vi "ExCamApp.vi"() -> ()   [LabVIEW 2010]
uses:
  MaxY.vi
  MaxX.vi
  temperture.vi
  Binning.vi
  ADC.vi
  readoutport.vi
panel:
  out "Boolean":bool
  in  "Leave Program":bool
  in  "Tab Control":T1(tab)
  out "Pixel Time":i32
  out "Bit Depth":i32
  out "ReadOut port":i32
  out "ADC Offset":i32
  out "ADC Gain":i32
  out "ADC Speed":i32
  in  "Set Controller Variables":bool
  in  "Readout Port":bool
  in  "Gain (0-3)":u32
  in  "ADC Rate":bool
  in  "OK Button 2":bool
  out "Current Temperature":dbl format="%.2f"
  in  "Temperature":dbl format="%.2f"
  out "Thermometer":dbl(slide) scale=-90.0..20.0
  out "End Y":u32=1 min=1 step=1
  out "Start Y":u32=1 min=1 step=1
  in  "OK Button 5":bool
  in  "OK Button 4":bool
  out "Bin Amount":u32
  in  "OK Button 3":bool
  in  "Exposure (sec)":dbl format="%.2f"
  in  "OK Button":bool
  out "Waveform Graph":sgl[](graph)
  out "Bin value":u32
  in  "OK Button 10":bool
  in  "OK Button 9":bool
  in  "OK Button 8":bool
  in  "OK Button 7":bool
  in  "Exposure (sec)":dbl format="%.2f"
  in  "OK Button 6":bool
  out "error out":errorcluster
  in  "error in (no error)":errorcluster
  # "Current ADC  settings"
  # "High Speed"
  # "Low Speed"
  # "Low Noise"
  # "High Capacity"
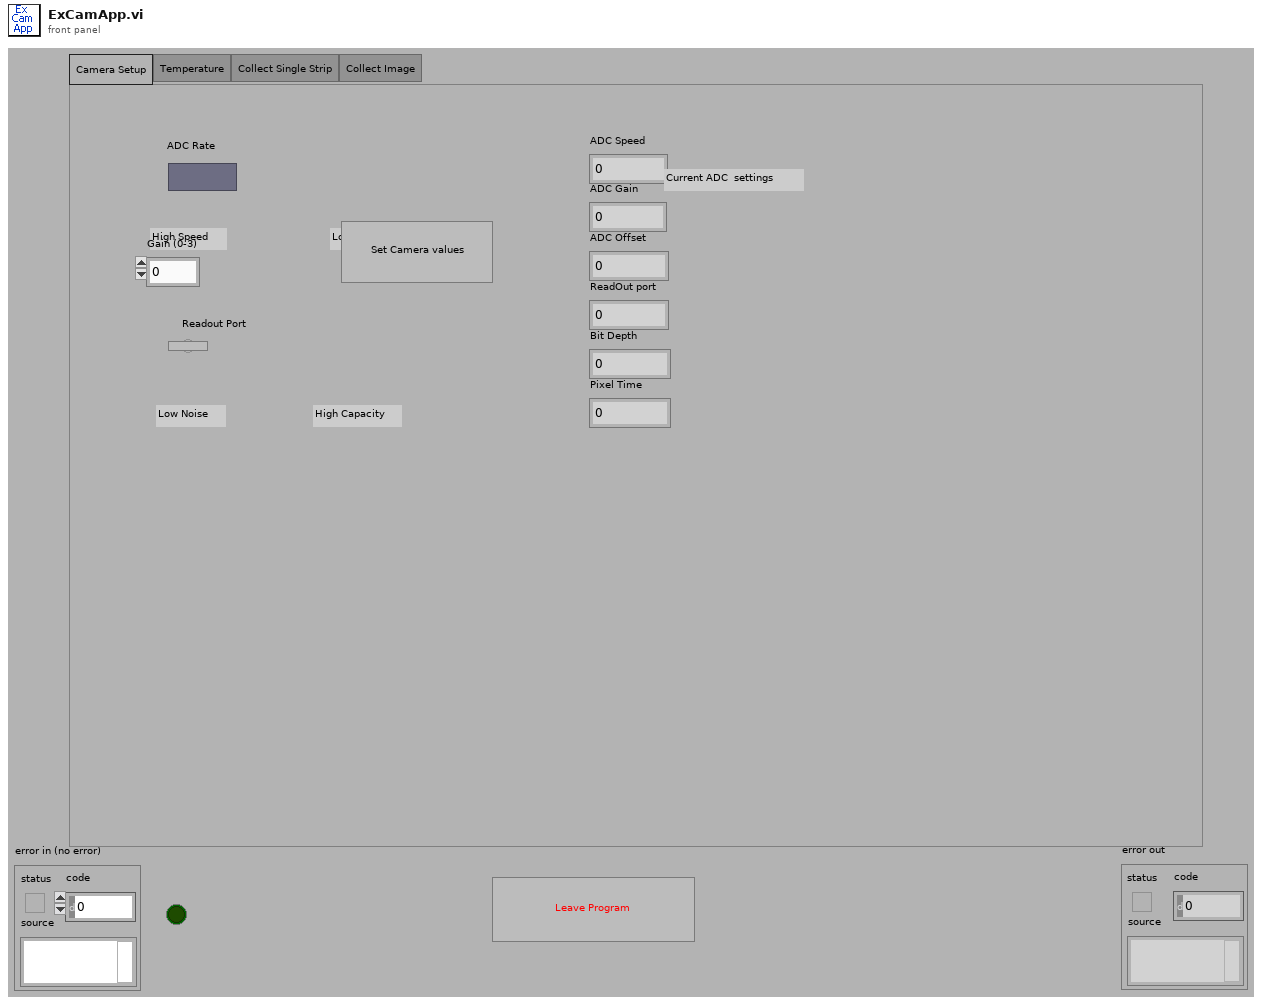
[diagram p1: front panel]
types:
  T1 = enum32{"Camera Setup", "Temperature", "Collect Single Strip", "Collect Image"}
  T2 = cluster{"X start":u32, "X end":u32, "X Binning/Grouping":u32, "Y start":u32, "Y end":u32, "Y Binning/Grouping":u32}
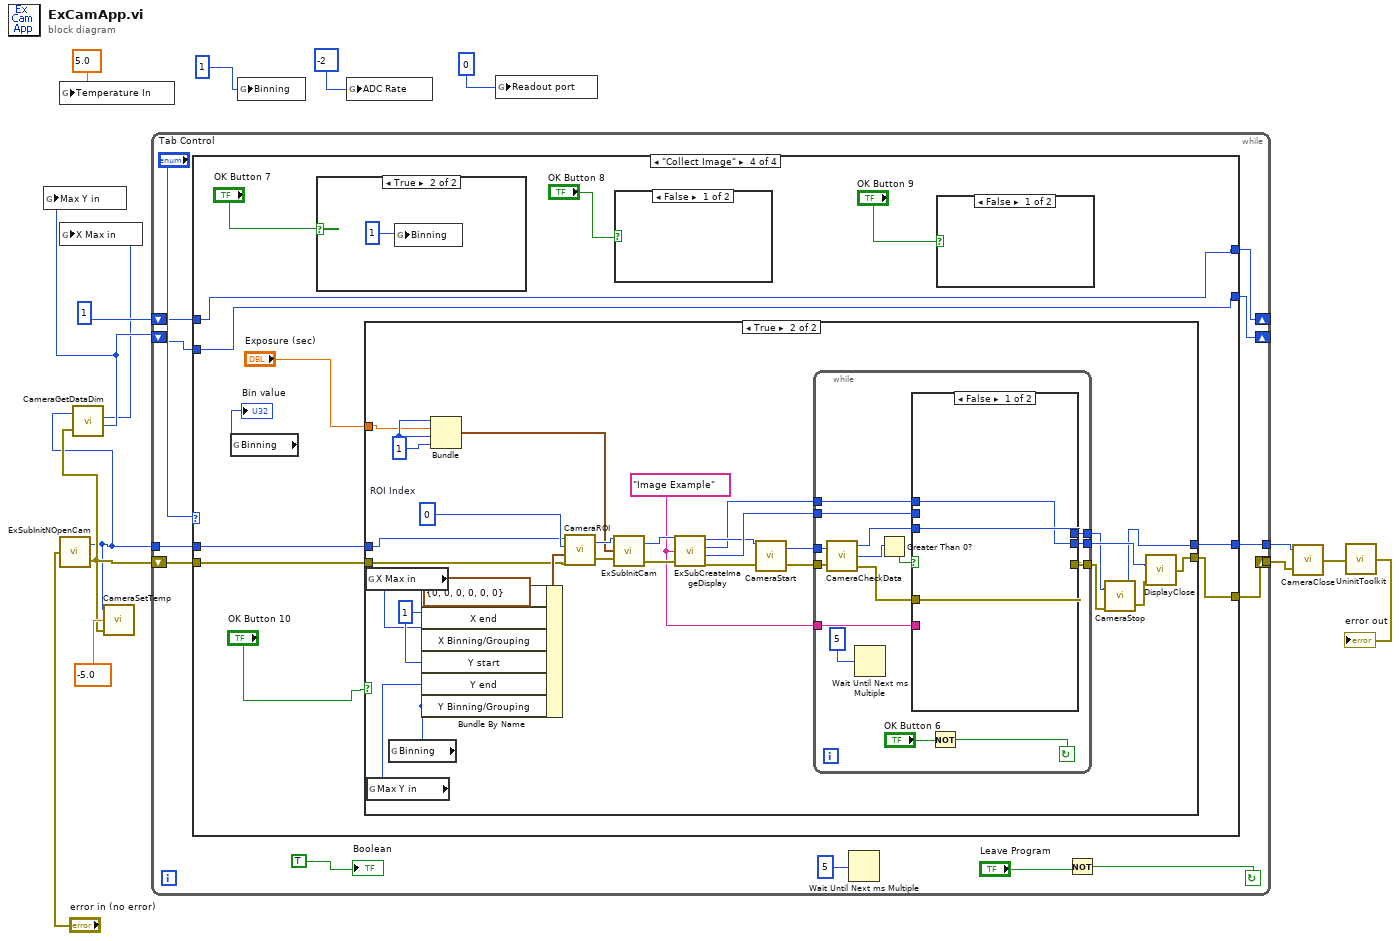
[diagram p0: block diagram]
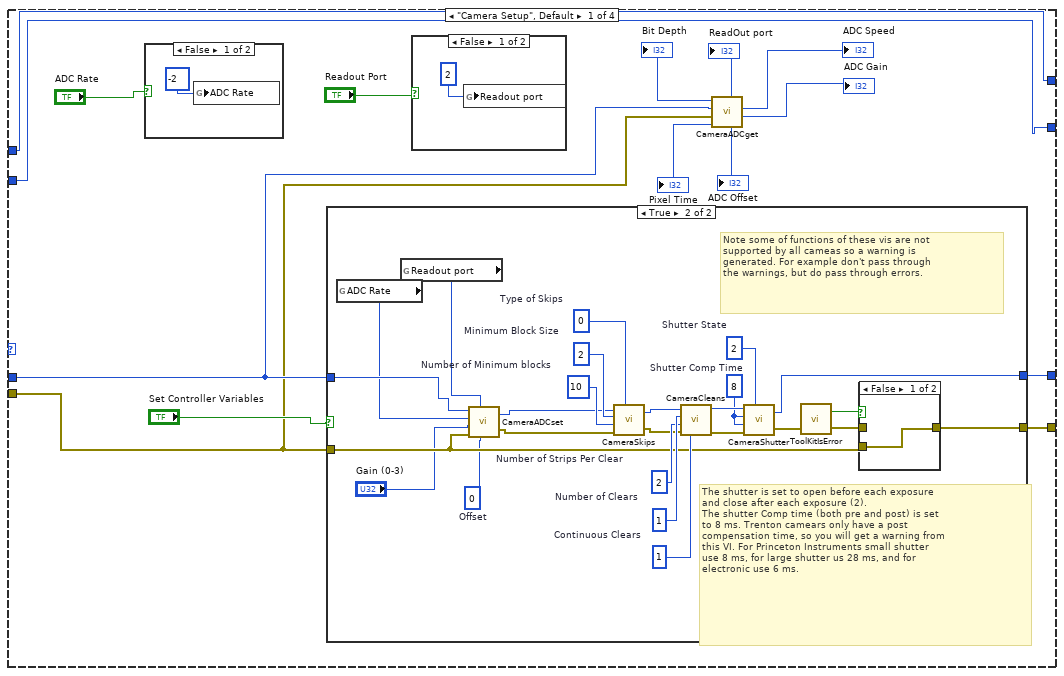
[diagram p2: hidden frame]
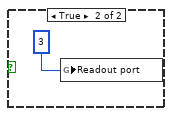
[diagram p3: hidden frame]
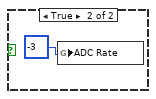
[diagram p4: hidden frame]
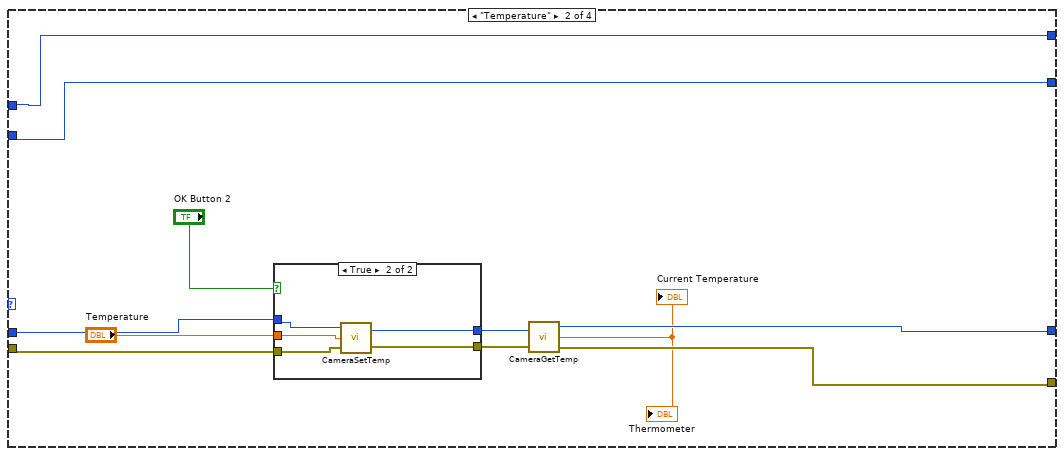
[diagram p7: hidden frame]
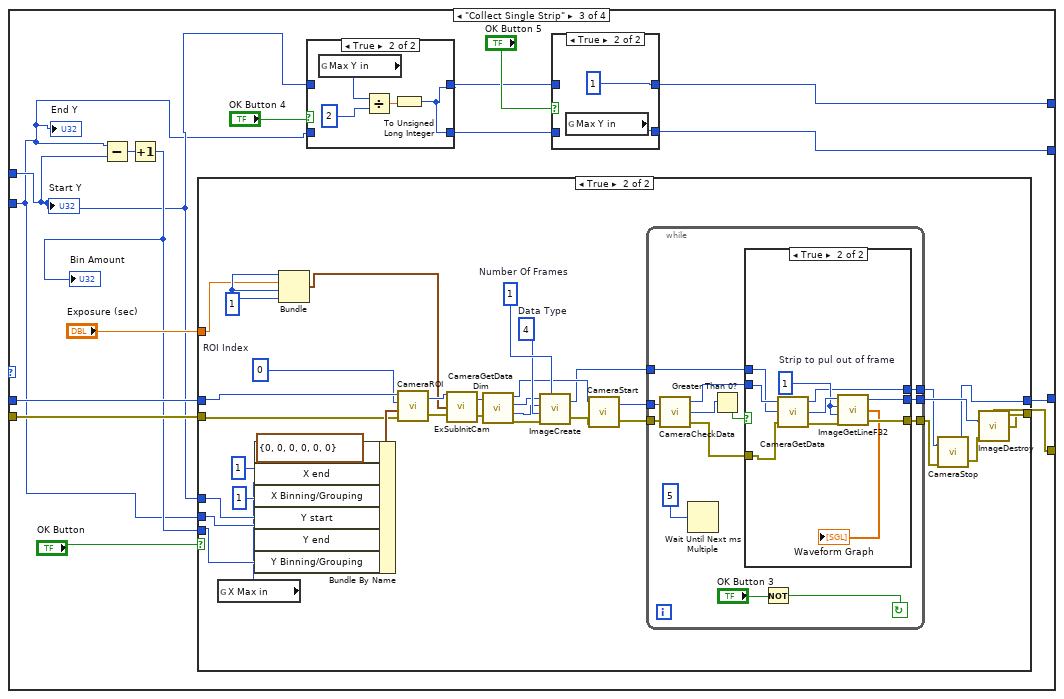
[diagram p9: hidden frame]
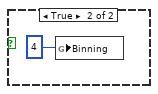
[diagram p14: hidden frame]
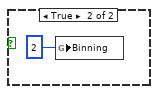
[diagram p15: hidden frame]
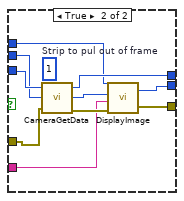
[diagram p18: hidden frame]
diagram:
  n1 = global write "temperture.vi" "Temperature In"(5.0) -> ()
  n2 = call "ExSubInitNOpenCam.vi"("error in (no error)"="error in (no error)") -> ("Camera Handle"=w1:u32, "error out"=w2:errorcluster)
  n3 = call <userlib>:"CameraGetDataDim.vi"("Camera Handle"=w1, "error in"=w2) -> ("Xdim"=w11:u32, "Ydim"=w12:u32)  [unwired: 2 out]
  n4 = global write "MaxY.vi" "Max Y in"(w12) -> ()
  n5 = global write "MaxX.vi" "X Max in"(w11) -> ()
  n6 = call <userlib>:"CameraSetTemp.vi"("error in (no error)"=w2, "Temperature"=-5.0, "Camera Handle"=w1) -> ()  [unwired: 2 out]
  n7 = while {
    shift-right: [w18] -> _
    shift-left: w2 -> [w26]
    tunnel: w1 -> [w27]
    shift-right: [w23] -> _
    shift-left: 1 -> [w25]
    shift-right: [w22] -> _
    shift-left: w12 -> [w24]
    tunnel: [w18] -> w10
    tunnel: [w17] -> w9
    stop <- w20 continue-if-true
    n8 = case shown="\"Collect Image\"" "Tab Control" {
      tunnel: [w43 w82 w97 w194] -> w18
      tunnel: w27 -> [w30 w87 w102 w191]
      tunnel: [w42 w81 w98 w193] -> w17
      tunnel: w26 -> [w29 w86 w101 w190]
      tunnel: w25 -> [w41 w79 w96 w185]
      tunnel: w24 -> [w40 w78 w95 w186]
      tunnel: [w41 w79 w104 w185] -> w23
      tunnel: [w40 w78 w103 w186] -> w22
      frame "Camera Setup", Default {
        n9 = case shown="False" "ADC Rate" {
          frame False {
            n10 = global write "ADC.vi" "ADC Rate"(-2) -> ()
          }
          frame True {
            n11 = global write "ADC.vi" "ADC Rate"(-3) -> ()
          }
        }
        n12 = case shown="True" "Set Controller Variables" {
          tunnel: [w48 w59] -> w43
          tunnel: w30 -> [w49 w54]
          tunnel: [w49 w58] -> w42
          tunnel: w29 -> [w48 w57]
          frame False {
          }
          frame True {
            w50 = 0  # Offset
            w66 = u32 0  # Type of Skips
            w67 = u32 2  # Minimum Block Size
            w65 = u32 10  # Number of Minimum blocks
            w69 = u32 1  # Number of Clears
            w68 = u32 2  # Number of Strips Per Clear
            w70 = u32 1  # Continuous Clears
            w71 = u32 2  # Shutter State
            w72 = u32 8  # Shutter Comp Time
            # "Note some of functions of these vis are not \nsupported by all cameas so a warning is \ngenerated. For example don't pass through \nthe warnings, but do pass through errors."
            # "The shutter is set to open before each exposure \nand close after each exposure (2).\nThe shutter Comp time (both pre and post) is set \nto 8 ms. Trenton camears only have a post \ncompensation time, so you will get a warning from \nthis VI. For Princeton Instruments small shutter \nuse 8 ms, for large shutter us 28 ms, and for \nelectronic use 6 ms."
            n13 = global read "ADC.vi" "ADC Rate"() -> (w52:i32)
            n14 = global read "readoutport.vi" "Readout port"() -> (w53:u32)
            n15 = call <userlib>:"CameraADCset.vi"("ADC offset"=w50, "Read Out port"=w53, "error in (no error)"=w57, "ADC Gain"="Gain (0-3)", "ADC Speed"=w52, "Camera Handle"=w54) -> ("error out"=w56:errorcluster, "Camera Handle"=w55:u32)
            n16 = call <userlib>:"CameraSkips.vi"("Camera Handle"=w55, "Minimum Block Size"=w67, "Number of Minimum blocks"=w65, "error in"=w56, "Type of Skips"=w66) -> ("Camera Handle"=w64:u32, "error out"=w63:errorcluster)
            n17 = call <userlib>:"CameraCleans.vi"("Camera Handle"=w64, "Number of Clears"=w69, "Number of Strips Per Clear"=w68, "error in"=w63, "Continuous Clears"=w70) -> ("Camera Handle"=w73:u32, "error out"=w74:errorcluster)
            n18 = call <userlib>:"CameraShutter.vi"("Camera Handle"=w73, "Shutter Comp Time: Pre Open"=w72, "Shutter Comp Time: Post Open"=w72, "error in"=w74, "Shutter State"=w71) -> ("Camera Handle"=w58:u32, "error out"=w62:errorcluster)
            n19 = call <userlib>:"ToolKitIsError.vi"("error in"=w62) -> ("error out"=w60:errorcluster, "Error Flag"=w61:bool)  [unwired: 1 in]
            n20 = case shown="False" w61 {
              tunnel: w60 -> [_ w76]
              tunnel: [w75 w76] -> w59
              tunnel: w57 -> [w75 _]
              frame False {
              }
              frame True {
              }
            }
          }
        }
        n21 = case shown="False" "Readout Port" {
          frame False {
            n22 = global write "readoutport.vi" "Readout port"(2) -> ()
          }
          frame True {
            n23 = global write "readoutport.vi" "Readout port"(3) -> ()
          }
        }
        n24 = call <userlib>:"CameraADCget.vi"("Camera handle"=w30, "error in (no error)"=w29) -> ("Bit Depth"=→"Bit Depth":i32, "Pixel Time"=→"Pixel Time":i32, "Readout Port"=→"ReadOut port":i32, "ADC Offset"=→"ADC Offset":i32, "ADC Speed"=→"ADC Speed":i32, "ADC Gain"=→"ADC Gain":i32)  [unwired: 2 out]
      }
      frame "Temperature" {
        n25 = case shown="True" "OK Button 2" {
          tunnel: w87 -> [w89 w94]
          tunnel: w86 -> [w88 w93]
          tunnel: "Temperature" -> [_ w90]
          tunnel: [w88 w92] -> w84
          tunnel: [w89 w91] -> w83
          frame False {
          }
          frame True {
            n26 = call <userlib>:"CameraSetTemp.vi"("error in (no error)"=w93, "Temperature"=w90, "Camera Handle"=w94) -> ("error out"=w92:errorcluster, "Camera Handle"=w91:u32)
          }
        }
        n27 = call <userlib>:"CameraGetTemp.vi"("Camera Handle"=w83, "error in (no error)"=w84) -> ("Camera Handle"=w81:u32, "Temperature"=→"Thermometer" →"Current Temperature":dbl, "error out"=w82:errorcluster)
      }
      frame "Collect Single Strip" {
        n28 = Subtract(x=w95, y=w96) -> (x-y=w109:u32)
        n29 = Increment(x=w109) -> (x+1=w99:u32)
        "Bin Amount" <- w99
        n30 = case shown="True" "OK Button" {
          tunnel: w102 -> [w122 w143]
          tunnel: [w122 w125] -> w98
          tunnel: w101 -> [w121 w144]
          tunnel: [w121 w128] -> w97
          tunnel: "Exposure (sec)" -> [_ w141]
          tunnel: w95 -> [_ w149]
          tunnel: w96 -> [_ w148]
          tunnel: w99 -> [_ w147]
          frame False {
          }
          frame True {
            w138 = u32 4  # Data Type
            w139 = u32 1  # Number Of Frames
            w142 = u32 0  # ROI Index
            w154 = 1
            n31 = global read "MaxX.vi" "X Max in"() -> (w146:u32)
            n32 = Bundle By Name(cluster=T2 {"X start"=0, "X end"=0, "X Binning/Grouping"=0, "Y start"=0, "Y end"=0, "Y Binning/Grouping"=0} ("ROI Params"), "X start"=u32 1, "X end"=w146, "X Binning/Grouping"=u32 1, "Y start"=w148, "Y end"=w149, "Y Binning/Grouping"=w147) -> (w145:T2)
            n33 = Bundle(w154, "Exposure (sec)"=w141, w154, w154) -> (w153:cluster{i32, "Exposure (sec)":dbl, i32, i32})  [unwired: 1 in]
            n34 = call <userlib>:"CameraROI.vi"("error in"=w144, "ROI Params"=w145, "ROI Index"=w142, "Camera Handle"=w143) -> ("error out"=w156:errorcluster, "Camera Handle"=w155:u32)
            n35 = call "ExSubInitCam.vi"("error in (no error)"=w156, "Camera Information"=w153, "Camera Handle"=w155) -> ("error out"=w137:errorcluster, "Camera Handle"=w136:u32)
            n36 = call <userlib>:"CameraGetDataDim.vi"("Camera Handle"=w136, "error in"=w137) -> ("Camera Handle"=w133:u32, "Xdim"=w134:u32, "Ydim"=w135:u32, "error out"=w140:errorcluster)
            n37 = call <userlib>:"ImageCreate.vi"("X dimension"=w134, "Y dimension"=w135, "Data Type"=w138, "error in"=w140, "Number Of Frames"=w139) -> ("Image Handle"=w129:u32, "error out"=w132:errorcluster)
            n38 = call <userlib>:"CameraStart.vi"("error in"=w132, "Camera Handle"=w133) -> ("error out"=w131:errorcluster, "Camera Handle"=w130:u32)
            n39 = while {
              tunnel: w131 -> [w167]
              tunnel: w130 -> [w165]
              tunnel: w129 -> [w164]
              tunnel: [w160] -> w126
              tunnel: [w159] -> w123
              tunnel: [w158] -> w127
              stop <- w168 continue-if-true
              n40 = call <userlib>:"CameraCheckData.vi"("Camera Handle"=w165, "error in"=w167) -> ("Camera Handle"=w161:u32, "Number Of Frames Available"=w163:i32, "error out"=w166:errorcluster)
              n41 = Wait Until Next ms Multiple(millisecond multiple=5) -> ()  [unwired: 1 out]
              n42 = Greater Than 0?(x=w163) -> (x > 0?=w162:bool)
              n43 = case shown="True" w162 {
                tunnel: w166 -> [w172 w179]
                tunnel: w164 -> [w170 w177]
                tunnel: w161 -> [w171 w178]
                tunnel: [w171 w176] -> w160
                tunnel: [w170 w175] -> w158
                tunnel: [w172 w174] -> w159
                frame False {
                }
                frame True {
                  w180 = 1  # Strip to pul out of frame
                  n44 = call <userlib>:"CameraGetData.vi"("error in"=w179, "Data Handle"=w177, "Camera Handle"=w178) -> ("error out"=w182:errorcluster, "Data Handle"=w181:u32, "Camera Handle"=w176:u32)
                  n45 = call <userlib>:"ImageGetLineF32.vi"("error in"=w182, "Z Position"=w180, "Y Position"=w180, "Data Handle"=w181) -> ("error out"=w174:errorcluster, "Array F32"=→"Waveform Graph":sgl[], "Data Handle"=w175:u32)
                }
              }
              n46 = Not(x="OK Button 3") -> (.not. x?=w168:bool)
            }
            n47 = call <userlib>:"CameraStop.vi"("error in"=w123, "Camera Handle"=w126) -> ("error out"=w124:errorcluster, "Camera Handle"=w125:u32)
            n48 = call <userlib>:"ImageDestroy.vi"("error in"=w124, "Data handle"=w127) -> ("error out"=w128:errorcluster)
          }
        }
        n49 = case shown="True" "OK Button 4" {
          tunnel: w96 -> [w116 _]
          tunnel: w95 -> [w115 _]
          tunnel: [w116 w117] -> w106
          tunnel: [w115 w117] -> w105
          frame False {
          }
          frame True {
            n50 = global read "MaxY.vi" "Max Y in"() -> (w119:u32)
            n51 = Divide(x=w119, y=2) -> (x/y=w118:dbl)
            n52 = To Unsigned Long Integer(number=w118) -> (unsigned 32bit integer=w117:u32)
          }
        }
        n53 = case shown="True" "OK Button 5" {
          tunnel: w106 -> [w112 _]
          tunnel: w105 -> [w111 _]
          tunnel: [w112 1] -> w104
          tunnel: [w111 w113] -> w103
          frame False {
          }
          frame True {
            n54 = global read "MaxY.vi" "Max Y in"() -> (w113:u32)
          }
        }
        "Start Y" <- w96
        "End Y" <- w95
      }
      frame "Collect Image" {
        n55 = global read "Binning.vi" "Binning"() -> (→"Bin value":u32)
        n56 = case shown="True" "OK Button 7" {
          frame False {
          }
          frame True {
            n57 = global write "Binning.vi" "Binning"(1) -> ()
          }
        }
        n58 = case shown="True" "OK Button 10" {
          tunnel: [w198 w215] -> w193
          tunnel: [w199 w218] -> w194
          tunnel: "Exposure (sec)" -> [_ w207]
          tunnel: w191 -> [w198 w205]
          tunnel: w190 -> [w199 w204]
          frame False {
          }
          frame True {
            w202 = "Image Example"
            w221 = u32 0  # ROI Index
            w225 = u32 1
            w226 = 1
            n59 = global read "MaxX.vi" "X Max in"() -> (w223:u32)
            n60 = global read "MaxY.vi" "Max Y in"() -> (w201:u32)
            n61 = global read "Binning.vi" "Binning"() -> (w200:u32)
            n62 = Bundle By Name(cluster=T2 {"X start"=0, "X end"=0, "X Binning/Grouping"=0, "Y start"=0, "Y end"=0, "Y Binning/Grouping"=0} ("ROI Params"), "X start"=w225, "X end"=w223, "X Binning/Grouping"=w200, "Y start"=w225, "Y end"=w201, "Y Binning/Grouping"=w200) -> (w222:T2)
            n63 = Bundle(w226, "Exposure (sec)"=w207, w226, w226) -> (w206:cluster{i32, "Exposure (sec)":dbl, i32, i32})  [unwired: 1 in]
            n64 = call <userlib>:"CameraROI.vi"("error in"=w204, "ROI Params"=w222, "ROI Index"=w221, "Camera Handle"=w205) -> ("error out"=w228:errorcluster, "Camera Handle"=w227:u32)
            n65 = call "ExSubInitCam.vi"("error in (no error)"=w228, "Camera Information"=w206, "Camera Handle"=w227) -> ("error out"=w212:errorcluster, "Camera Handle"=w208:u32)
            n66 = call "ExSubCreateImageDisplay.vi"("Camera Handle"=w208, "File and Display Name"=w202, "error in (no error)"=w212) -> ("Camera Handle"=w209:u32, "Display Handle"=w203:u32, "Image Handle"=w210:u32, "error out"=w211:errorcluster)
            n67 = call <userlib>:"CameraStart.vi"("error in"=w211, "Camera Handle"=w209) -> ("error out"=w220:errorcluster, "Camera Handle"=w219:u32)
            n68 = while {
              tunnel: w220 -> [w241]
              tunnel: w219 -> [w239]
              tunnel: w210 -> [w238]
              tunnel: [w234] -> w216
              tunnel: [w233] -> w213
              tunnel: [w232] -> w217
              tunnel: w203 -> [w230]
              tunnel: w202 -> [w229]
              stop <- w242 continue-if-true
              n69 = call <userlib>:"CameraCheckData.vi"("Camera Handle"=w239, "error in"=w241) -> ("Camera Handle"=w235:u32, "Number Of Frames Available"=w237:i32, "error out"=w240:errorcluster)
              n70 = Wait Until Next ms Multiple(millisecond multiple=5) -> ()  [unwired: 1 out]
              n71 = Greater Than 0?(x=w237) -> (x > 0?=w236:bool)
              n72 = case shown="False" w236 {
                tunnel: w240 -> [w246 w256]
                tunnel: w238 -> [_ w254]
                tunnel: w235 -> [w245 w255]
                tunnel: [w245 w253] -> w234
                tunnel: [w244 w250] -> w232
                tunnel: [w246 w251] -> w233
                tunnel: w230 -> [w244 w248]
                tunnel: w229 -> [_ w247]
                frame False {
                }
                frame True {
                  (unwired) 1  # Strip to pul out of frame
                  n73 = call <userlib>:"CameraGetData.vi"("error in"=w256, "Data Handle"=w254, "Camera Handle"=w255) -> ("error out"=w252:errorcluster, "Data Handle"=w249:u32, "Camera Handle"=w253:u32)
                  n74 = call <userlib>:"DisplayImage.vi"("error in"=w252, "Title"=w247, "Image Handle"=w249, "Display Handle"=w248) -> ("error out"=w251:errorcluster, "Display Handle"=w250:u32)
                }
              }
              n75 = Not(x="OK Button 6") -> (.not. x?=w242:bool)
            }
            n76 = call <userlib>:"CameraStop.vi"("error in"=w213, "Camera Handle"=w216) -> ("error out"=w214:errorcluster, "Camera Handle"=w215:u32)
            n77 = call <userlib>:"DisplayClose.vi"("error in"=w214, "Display Handle"=w217) -> ("error out"=w218:errorcluster)
          }
        }
        n78 = case shown="False" "OK Button 8" {
          frame False {
          }
          frame True {
            n79 = global write "Binning.vi" "Binning"(2) -> ()
          }
        }
        n80 = case shown="False" "OK Button 9" {
          frame False {
          }
          frame True {
            n81 = global write "Binning.vi" "Binning"(4) -> ()
          }
        }
      }
    }
    n82 = Wait Until Next ms Multiple(millisecond multiple=5) -> ()  [unwired: 1 out]
    n83 = Not(x="Leave Program") -> (.not. x?=w20:bool)
    "Boolean" <- TRUE
  }
  n84 = global write "Binning.vi" "Binning"(1) -> ()
  n85 = global write "ADC.vi" "ADC Rate"(-2) -> ()
  n86 = global write "readoutport.vi" "Readout port"(0) -> ()
  n87 = call <userlib>:"CameraClose.vi"("error in"=w10, "Camera Handle"=w9) -> ("error out"=w8:errorcluster)
  n88 = call <userlib>:"UninitToolkit.vi"("error in"=w8) -> ("error out"=→"error out":errorcluster)
